vi "Wait for VI loaded.vi"(8 "error in":errorcluster, 9 "timeout min [sec]":dbl=2.0, 10 "timeout max [sec]":dbl=10.0, 11 "VI Referenz":refnum<vi>) -> (0 "error out":errorcluster, 2 "timed out":bool, 3 "VI Referenz out":refnum<vi>)   [LabVIEW 2020, in "Backup.lvlib"]
doc: "Wartet bis die angegebene VI Referenze im Status \"idle\" läuft,\noder timeout max (in sec) eintritt (Default sind 10 sec) - dann wird \"timed out\" gesetzt\nund mindestens timeout min (in sec, Default ist 2 sec) erreicht wurde,\num sicher zu stellen, dass das VI vollständig geladen wurde,\num Werte abzufrgen oder einen ScreeShot zu machen ...\nriw 04.02.2019"
uses:
  Backup.lvlib
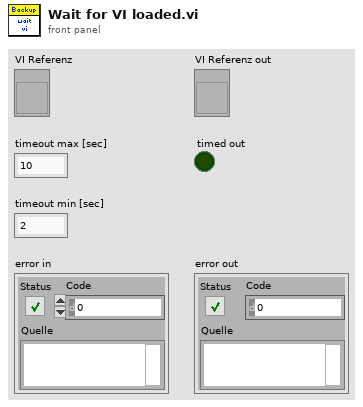
[diagram p1: front panel]
types:
  T1 = enum32{"Bad", "Idle", "Run top level", "Running"}
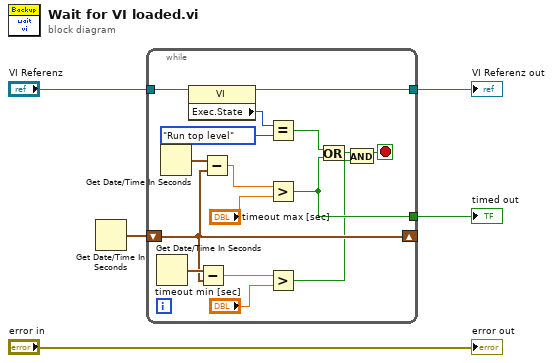
[diagram p0: block diagram]
diagram:
  n1 = Get Date/Time In Seconds() -> (seconds since 1Jan1904=w3:timestamp)
  n2 = while {
    tunnel: "VI Referenz" -> [w21]
    shift-right: [w10] -> _
    shift-left: w3 -> [w10]
    tunnel: [w13] -> w2
    tunnel: [w12] -> w1
    stop <- w7 stop-if-true
    n3 = Get Date/Time In Seconds() -> (seconds since 1Jan1904=w11:timestamp)
    n4 = Get Date/Time In Seconds() -> (seconds since 1Jan1904=w17:timestamp)
    n5 = property class="VI"(reference=w21) -> (reference out=w13:refnum<vi>, "Exec.State"=w19:T1)  [unwired: 1 in, 1 out]
    n6 = Subtract(x=w11, y=w10) -> (x-y=w8:dbl)
    n7 = Subtract(x=w17, y=w10) -> (x-y=w16:dbl)
    n8 = Equal?(x=w19, y=T1."Run top level" ("Ausführung:Status")) -> (x = y?=w20:bool)
    n9 = Greater?(x=w16, y="timeout max [sec]") -> (0:w12:bool)
    n10 = Greater?(x=w8, y="timeout min [sec]") -> (0:w6:bool)
    n11 = Or(x=w20, y=w12) -> (x .or. y?=w15:bool)
    n12 = And(x=w15, y=w6) -> (x .and. y?=w7:bool)
  }
  "VI Referenz out" <- w2
  "timed out" <- w1
  "error out" <- "error in"
